vi "MNIST_weight_2color_print_sub.vi"(1 "최소값":dbl=-2.4903133, 2 "최대값":dbl=1.9686242, 3 "배열":dbl[][](array[numeric])=[[0.06671473, 0.012806132, 0.0, 0.007022038, 0.075053, 0.052519154, 0.06788373, 0.058529492, 0.068049595, 0.005657882, 0.0, 0.019000702, 0.10409468, 0.038491603, 0.0, 0.0, 0.0, 0.0, 0.0, 0.0, 0.029719673, 0.0589787, 0.012006044, 0.0, 0.0, 0.0, 0.003024332, 0.0], [0.046028584, 0.084819525, 0.0, 0.0, 0.0, 0.0, 0.027638003, 0.11720828, 0.1663973, 0.25961968, 0.31170687, 0.5143633, 0.3731328, 0.48274365, 0.3280385, 0.40694475, 0.35356778, 0.38455793, 0.24461184, 0.29286602, 0.4148841, 0.408167, 0.36261445, 0.4037632, 0.013449289, 0.07692665, 0.0, 0.028387021], [0.003123008, 0.07717365, 0.07922222, 0.3189904, 0.28332156, 0.062017616, 0.13301574, 0.2924652, 0.2965881, 0.29845756, 0.5972768, 0.6319597, 0.66892195, 0.64722604, 0.62055475, 0.6523688, 0.6531713, 0.83753306, 0.55209464, 0.5967644, 0.49876857, 0.44684905, 0.4477752, 0.5052764, 0.0, 0.0, 0.05617176, 0.020920113], [0.024063304, 0.056840383, 0.0, 0.39337757, 0.30629715, 0.37364787, 0.34470925, 0.5042887, 0.4251124, 0.506105, 0.89726394, 1.1779351, 1.5517938, 1.5492246, 1.8865724, 1.8361284, 1.6005924, 0.8755611, 0.17848553, 0.19548813, 0.6069504, 0.6787907, 0.27294815, 0.20360427, 0.16959353, 0.022720885, 0.0, 0.004873298], [0.08592967, 0.06972434, 0.0, 0.25001055, 0.006792835, 0.4052463, 0.57627326, 1.0514435, 1.1154656, 1.5954032, 1.678078, 0.962688, 0.9687104, 0.89993167, 0.7828392, 1.0242023, 1.1486256, 1.0977578, 0.95435023, 2.3045535, 2.3393528, 2.0629787, 1.3075817, 1.1000681, 0.6505148, 0.15433559, 0.12817676, 0.07914265], [0.07988503, 0.0, 0.0, 0.31504992, 0.37430423, 0.88769066, 1.5406835, 0.6172341, 0.29620916, 0.47488296, 0.26253828, 0.0, 0.0, 0.0, 0.19108367, 0.08104278, 0.515581, 0.37645754, 0.33281028, 0.25179097, 0.22456875, 0.4467277, 0.6797482, 2.2890959, 1.863171, 0.833423, 0.43375036, 0.10676513], [0.0, 0.21307647, 0.5049865, 0.45892584, 0.85746795, 1.20627, 0.48567757, 0.30300915, 0.2370981, 0.0, 0.0, 0.0, 0.0, 0.0, 0.0, 0.0, 0.0, 0.0, 0.0, 0.0, 0.0, 0.054976966, 0.33023435, 0.74540865, 0.82584643, 0.3999863, 0.7573047, 0.37040982], [0.0, 0.48237345, 0.60469353, 0.83249414, 1.066871, 0.8326912, 0.3114878, 0.39401188, 0.03141666, 0.0, 0.0, 0.0, 0.0, 0.0, 0.0, 0.0, 0.0, 0.0, 0.0, 0.0, 0.0, 0.0, 0.1001043, 0.222988, 0.7484905, 0.8096203, 0.9580958, 0.50581247], [0.23312153, 0.81503505, 0.93997633, 0.89034003, 0.5627975, 0.27621332, 0.0881613, 0.30927205, 0.0, 0.0990191, 0.040483538, 0.15247008, 0.17033584, 0.0, 0.0, 0.0, 0.0, 0.0, 0.0, 0.0, 0.095491596, 0.0, 0.15988904, 0.4184175, 0.5088815, 0.7918951, 0.9527885, 0.27583468], [0.34983167, 0.5911077, 1.0430478, 0.4566845, 0.40939477, 0.05266172, 0.0, 0.0, 0.0, 0.02691007, 0.0, 0.016026955, 0.0, 0.0, 0.0, 0.0, 0.009803846, 0.0, 0.0, 0.04322388, 0.032798484, 0.23765023, 0.17197067, 0.44923514, 0.4066683, 0.8139697, 0.9593992, 0.4893604], [0.2907163, 0.5717058, 1.0163774, 0.38863152, 0.29278657, 0.0, 0.0, 0.0, 0.0, 0.0, 0.0, 0.0, 0.0, 0.14446034, 0.09155477, 0.14909427, 0.024265863, 0.0, 0.0, 0.06254616, 6.79e-05, 0.082516626, 0.13715447, 0.32466382, 0.7280415, 0.36880082, 0.9140208, 0.4657428], [0.33525127, 0.6217594, 0.82226497, 0.44135088, 0.16826938, 0.0, 0.0, 0.0, 0.0, 0.0, 0.0, 0.0, 0.011187709, 0.11938254, 0.015615412, 0.0, 0.0, 0.0, 0.0, 0.0, 0.0, 0.0, 0.0, 0.2770026, 0.6325938, 0.631355, 0.6114226, 0.3128235], [0.22835304, 0.7955853, 0.71307003, 0.35154894, 0.0, 0.0, 0.0, 0.0, 0.0, 0.0, 0.0, 0.0, 0.2698419, 0.0, 0.0, 0.0, 0.0, 0.0, 0.0, 0.0, 0.0, 0.0, 0.0, 0.0, 1.0116065, 1.7317381, 0.8858002, 0.3161338], [0.18020941, 0.53125805, 0.6827323, 0.21136676, 0.0, 0.0, 0.0, 0.0, 0.0, 0.0, 0.0, 0.055699844, 0.27314368, 0.0, 0.0, 0.0, 0.0, 0.0, 0.0, 0.0, 0.0, 0.0, 0.0, 0.29844484, 1.5662781, 1.1574728, 0.55202866, 0.085822225], [0.31430015, 0.3546583, 0.7948181, 0.0, 0.0, 0.058352455, 0.0, 0.0, 0.0, 0.0, 0.0, 0.051398423, 0.12864865, 0.0, 0.0, 0.0, 0.0, 0.0, 0.0, 0.0, 0.0, 0.0, 0.016005708, 0.70366126, 1.9256966, 0.7303306, 0.322807, 0.04477008], [0.2970737, 0.0, 0.9035585, 0.04951164, 0.001701124, 0.0, 0.0, 0.009708367, 0.0, 0.09480543, 0.0, 0.0, 0.07521264, 0.11005654, 0.10118085, 0.0, 0.0, 0.0, 0.0, 0.0, 0.0, 0.003710072, 0.018180061, 0.6137533, 1.6424786, 0.8153885, 0.11793761, 0.3056317], [0.29503796, 0.17651856, 0.58721036, 0.18996832, 0.008066228, 0.0, 0.15021098, 0.0, 0.0, 0.18720058, 0.0, 0.0, 0.05664227, 0.12680227, 0.091266185, 0.0, 0.0, 0.0, 0.0, 0.14982839, 0.15584202, 0.2898715, 0.03922329, 0.4780351, 1.6513777, 1.2352444, 0.48265705, 0.5113582], [0.042506717, 0.319817, 0.5209567, 0.3233532, 0.53686345, 0.36480454, 0.19566067, 0.0, 0.0, 0.0, 0.0, 0.0, 0.0, 0.09237474, 0.010339986, 0.0, 0.0, 0.0, 0.012240005, 0.04897488, 0.14640339, 0.19739835, 0.28918922, 0.5824203, 1.4695345, 0.6496217, 0.4080505, 0.47764888], [0.0, 0.2749003, 0.5060507, 0.59561384, 0.82417494, 0.56122655, 0.13255721, 0.04494526, 0.08564969, 0.16170388, 0.0, 0.0, 0.28955424, 0.25209564, 0.0, 0.0, 0.07394005, 0.0, 0.16412586, 0.12713751, 0.0417476, 0.2978168, 0.27767536, 0.7567341, 1.5418999, 0.675374, 0.66687757, 0.3468876], [0.0, 0.41774225, 1.0719318, 0.5180834, 0.65000916, 0.48373982, 0.18409592, 0.0, 0.18066232, 0.44167724, 0.21451446, 0.3340605, 0.2556067, 0.14536966, 0.17981717, 0.17562614, 0.12162264, 0.16115464, 0.23022401, 0.05762116, 0.051491685, 0.2887901, 0.37232834, 0.5140671, 0.8623661, 0.37336326, 0.38255432, 0.26215634], [0.083229735, 0.32688043, 0.608484, 0.41744143, 0.35103565, 0.22907315, 0.3805041, 0.46601966, 0.22916281, 0.5590473, 0.7263584, 0.6074327, 0.49197128, 0.24120732, 0.25589103, 0.28733763, 0.14443557, 0.14488553, 0.30391267, 0.15375902, 0.2781434, 0.5131602, 0.28703067, 0.30208346, 0.0, 0.0, 0.4837919, 0.002000345], [0.0, 0.32385758, 0.6328315, 0.80099195, 0.09775448, 0.07027386, 0.28887808, 0.2724674, 0.1625694, 0.0911344, 0.17027673, 0.32092783, 0.3155498, 0.26486373, 0.20463067, 0.17560713, 0.17749313, 0.29315472, 0.30376917, 0.29634923, 0.20721531, 0.13367781, 0.3279665, 0.28131253, 0.0, 0.020289743, 0.46843135, 0.027426496], [0.023119988, 0.06934198, 0.8942446, 0.27544105, 0.0, 0.28844702, 0.2773134, 0.26331362, 0.0, 0.0, 0.0, 0.0, 0.0, 0.075903945, 0.0, 0.22662191, 0.09397208, 0.24400133, 0.3108672, 0.43392682, 0.11429301, 0.15109178, 0.0, 0.0, 0.0, 0.030385807, 0.6572772, 0.0], [0.0, 0.0, 0.6131038, 0.18363582, 0.53004444, 0.26058108, 0.3353729, 0.16197264, 0.0, 0.1378254, 0.0, 0.054289043, 0.04886698, 0.07301120999999999, 0.004955645, 0.09871276, 0.16584411, 0.08512352, 0.16866887, 0.067276314, 0.0, 0.0, 0.0, 0.0, 0.0, 0.3628522, 0.4819391, 0.07737013], [0.0, 0.0, 0.39253348, 0.7897061, 0.08062354, 0.0, 0.0, 0.0, 0.0, 0.26711848, 0.03603759, 0.21447945, 0.15494835, 0.31901473, 0.26902923, 0.05804711, 0.076432385, 0.0, 0.01643955, 0.047397494, 0.0, 0.0, 0.0, 0.0, 0.23149125, 0.5096788, 0.36468777, 0.001521751], [0.0, 0.0, 0.0, 0.79396546, 0.0, 0.0, 0.0, 0.0, 0.0, 0.0, 0.0, 0.0, 0.0, 0.0, 0.0, 0.0, 0.0, 0.0, 0.0, 0.0, 0.0, 0.0, 0.009036388, 0.0, 0.26618186, 0.32190132, 0.31863904, 0.017361872], [0.041013133, 0.0, 0.012243457, 0.0, 0.0, 0.0, 0.0, 0.0, 0.0, 0.0, 0.0, 0.0, 0.0, 0.0, 0.0, 0.0, 0.0, 0.0, 0.0, 0.0, 0.0, 0.0, 0.0, 0.0, 0.0, 0.17493449, 0.0, 0.070362106], [0.022377841, 0.0, 0.07457931, 0.0, 0.4583214, 0.47468448, 0.0, 0.0, 0.0, 0.0, 0.0, 0.004390556, 0.0, 0.81566125, 0.0, 0.018186547, 0.18291555, 0.5620862, 0.06693945, 0.33189088, 0.0, 0.16514577, 0.3425562, 0.43024477, 0.0, 0.069507696, 0.0, 0.039162096], [0.3611892, 0.0, 0.0, 0.0, 0.0, 0.0, 0.0, 0.0, 0.0, 0.0, 0.0, 0.0, 0.0, 0.0, 0.0, 0.0, 0.0, 0.0, 0.0, 0.0, 0.0, 0.0, 0.0, 0.0, 0.0, 0.0, 0.0, 0.0]]) -> (0 "MNIST_Input":dbl[][](graph)=[[0.06671473, 0.012806132, 0.0, 0.007022038, 0.075053, 0.052519154, 0.06788373, 0.058529492, 0.068049595, 0.005657882, 0.0, 0.019000702, 0.10409468, 0.038491603, 0.0, 0.0, 0.0, 0.0, 0.0, 0.0, 0.029719673, 0.0589787, 0.012006044, 0.0, 0.0, 0.0, 0.003024332, 0.0], [0.046028584, 0.084819525, 0.0, 0.0, 0.0, 0.0, 0.027638003, 0.11720828, 0.1663973, 0.25961968, 0.31170687, 0.5143633, 0.3731328, 0.48274365, 0.3280385, 0.40694475, 0.35356778, 0.38455793, 0.24461184, 0.29286602, 0.4148841, 0.408167, 0.36261445, 0.4037632, 0.013449289, 0.07692665, 0.0, 0.028387021], [0.003123008, 0.07717365, 0.07922222, 0.3189904, 0.28332156, 0.062017616, 0.13301574, 0.2924652, 0.2965881, 0.29845756, 0.5972768, 0.6319597, 0.66892195, 0.64722604, 0.62055475, 0.6523688, 0.6531713, 0.83753306, 0.55209464, 0.5967644, 0.49876857, 0.44684905, 0.4477752, 0.5052764, 0.0, 0.0, 0.05617176, 0.020920113], [0.024063304, 0.056840383, 0.0, 0.39337757, 0.30629715, 0.37364787, 0.34470925, 0.5042887, 0.4251124, 0.506105, 0.89726394, 1.1779351, 1.5517938, 1.5492246, 1.8865724, 1.8361284, 1.6005924, 0.8755611, 0.17848553, 0.19548813, 0.6069504, 0.6787907, 0.27294815, 0.20360427, 0.16959353, 0.022720885, 0.0, 0.004873298], [0.08592967, 0.06972434, 0.0, 0.25001055, 0.006792835, 0.4052463, 0.57627326, 1.0514435, 1.1154656, 1.5954032, 1.678078, 0.962688, 0.9687104, 0.89993167, 0.7828392, 1.0242023, 1.1486256, 1.0977578, 0.95435023, 2.3045535, 2.3393528, 2.0629787, 1.3075817, 1.1000681, 0.6505148, 0.15433559, 0.12817676, 0.07914265], [0.07988503, 0.0, 0.0, 0.31504992, 0.37430423, 0.88769066, 1.5406835, 0.6172341, 0.29620916, 0.47488296, 0.26253828, 0.0, 0.0, 0.0, 0.19108367, 0.08104278, 0.515581, 0.37645754, 0.33281028, 0.25179097, 0.22456875, 0.4467277, 0.6797482, 2.2890959, 1.863171, 0.833423, 0.43375036, 0.10676513], [0.0, 0.21307647, 0.5049865, 0.45892584, 0.85746795, 1.20627, 0.48567757, 0.30300915, 0.2370981, 0.0, 0.0, 0.0, 0.0, 0.0, 0.0, 0.0, 0.0, 0.0, 0.0, 0.0, 0.0, 0.054976966, 0.33023435, 0.74540865, 0.82584643, 0.3999863, 0.7573047, 0.37040982], [0.0, 0.48237345, 0.60469353, 0.83249414, 1.066871, 0.8326912, 0.3114878, 0.39401188, 0.03141666, 0.0, 0.0, 0.0, 0.0, 0.0, 0.0, 0.0, 0.0, 0.0, 0.0, 0.0, 0.0, 0.0, 0.1001043, 0.222988, 0.7484905, 0.8096203, 0.9580958, 0.50581247], [0.23312153, 0.81503505, 0.93997633, 0.89034003, 0.5627975, 0.27621332, 0.0881613, 0.30927205, 0.0, 0.0990191, 0.040483538, 0.15247008, 0.17033584, 0.0, 0.0, 0.0, 0.0, 0.0, 0.0, 0.0, 0.095491596, 0.0, 0.15988904, 0.4184175, 0.5088815, 0.7918951, 0.9527885, 0.27583468], [0.34983167, 0.5911077, 1.0430478, 0.4566845, 0.40939477, 0.05266172, 0.0, 0.0, 0.0, 0.02691007, 0.0, 0.016026955, 0.0, 0.0, 0.0, 0.0, 0.009803846, 0.0, 0.0, 0.04322388, 0.032798484, 0.23765023, 0.17197067, 0.44923514, 0.4066683, 0.8139697, 0.9593992, 0.4893604], [0.2907163, 0.5717058, 1.0163774, 0.38863152, 0.29278657, 0.0, 0.0, 0.0, 0.0, 0.0, 0.0, 0.0, 0.0, 0.14446034, 0.09155477, 0.14909427, 0.024265863, 0.0, 0.0, 0.06254616, 6.79e-05, 0.082516626, 0.13715447, 0.32466382, 0.7280415, 0.36880082, 0.9140208, 0.4657428], [0.33525127, 0.6217594, 0.82226497, 0.44135088, 0.16826938, 0.0, 0.0, 0.0, 0.0, 0.0, 0.0, 0.0, 0.011187709, 0.11938254, 0.015615412, 0.0, 0.0, 0.0, 0.0, 0.0, 0.0, 0.0, 0.0, 0.2770026, 0.6325938, 0.631355, 0.6114226, 0.3128235], [0.22835304, 0.7955853, 0.71307003, 0.35154894, 0.0, 0.0, 0.0, 0.0, 0.0, 0.0, 0.0, 0.0, 0.2698419, 0.0, 0.0, 0.0, 0.0, 0.0, 0.0, 0.0, 0.0, 0.0, 0.0, 0.0, 1.0116065, 1.7317381, 0.8858002, 0.3161338], [0.18020941, 0.53125805, 0.6827323, 0.21136676, 0.0, 0.0, 0.0, 0.0, 0.0, 0.0, 0.0, 0.055699844, 0.27314368, 0.0, 0.0, 0.0, 0.0, 0.0, 0.0, 0.0, 0.0, 0.0, 0.0, 0.29844484, 1.5662781, 1.1574728, 0.55202866, 0.085822225], [0.31430015, 0.3546583, 0.7948181, 0.0, 0.0, 0.058352455, 0.0, 0.0, 0.0, 0.0, 0.0, 0.051398423, 0.12864865, 0.0, 0.0, 0.0, 0.0, 0.0, 0.0, 0.0, 0.0, 0.0, 0.016005708, 0.70366126, 1.9256966, 0.7303306, 0.322807, 0.04477008], [0.2970737, 0.0, 0.9035585, 0.04951164, 0.001701124, 0.0, 0.0, 0.009708367, 0.0, 0.09480543, 0.0, 0.0, 0.07521264, 0.11005654, 0.10118085, 0.0, 0.0, 0.0, 0.0, 0.0, 0.0, 0.003710072, 0.018180061, 0.6137533, 1.6424786, 0.8153885, 0.11793761, 0.3056317], [0.29503796, 0.17651856, 0.58721036, 0.18996832, 0.008066228, 0.0, 0.15021098, 0.0, 0.0, 0.18720058, 0.0, 0.0, 0.05664227, 0.12680227, 0.091266185, 0.0, 0.0, 0.0, 0.0, 0.14982839, 0.15584202, 0.2898715, 0.03922329, 0.4780351, 1.6513777, 1.2352444, 0.48265705, 0.5113582], [0.042506717, 0.319817, 0.5209567, 0.3233532, 0.53686345, 0.36480454, 0.19566067, 0.0, 0.0, 0.0, 0.0, 0.0, 0.0, 0.09237474, 0.010339986, 0.0, 0.0, 0.0, 0.012240005, 0.04897488, 0.14640339, 0.19739835, 0.28918922, 0.5824203, 1.4695345, 0.6496217, 0.4080505, 0.47764888], [0.0, 0.2749003, 0.5060507, 0.59561384, 0.82417494, 0.56122655, 0.13255721, 0.04494526, 0.08564969, 0.16170388, 0.0, 0.0, 0.28955424, 0.25209564, 0.0, 0.0, 0.07394005, 0.0, 0.16412586, 0.12713751, 0.0417476, 0.2978168, 0.27767536, 0.7567341, 1.5418999, 0.675374, 0.66687757, 0.3468876], [0.0, 0.41774225, 1.0719318, 0.5180834, 0.65000916, 0.48373982, 0.18409592, 0.0, 0.18066232, 0.44167724, 0.21451446, 0.3340605, 0.2556067, 0.14536966, 0.17981717, 0.17562614, 0.12162264, 0.16115464, 0.23022401, 0.05762116, 0.051491685, 0.2887901, 0.37232834, 0.5140671, 0.8623661, 0.37336326, 0.38255432, 0.26215634], [0.083229735, 0.32688043, 0.608484, 0.41744143, 0.35103565, 0.22907315, 0.3805041, 0.46601966, 0.22916281, 0.5590473, 0.7263584, 0.6074327, 0.49197128, 0.24120732, 0.25589103, 0.28733763, 0.14443557, 0.14488553, 0.30391267, 0.15375902, 0.2781434, 0.5131602, 0.28703067, 0.30208346, 0.0, 0.0, 0.4837919, 0.002000345], [0.0, 0.32385758, 0.6328315, 0.80099195, 0.09775448, 0.07027386, 0.28887808, 0.2724674, 0.1625694, 0.0911344, 0.17027673, 0.32092783, 0.3155498, 0.26486373, 0.20463067, 0.17560713, 0.17749313, 0.29315472, 0.30376917, 0.29634923, 0.20721531, 0.13367781, 0.3279665, 0.28131253, 0.0, 0.020289743, 0.46843135, 0.027426496], [0.023119988, 0.06934198, 0.8942446, 0.27544105, 0.0, 0.28844702, 0.2773134, 0.26331362, 0.0, 0.0, 0.0, 0.0, 0.0, 0.075903945, 0.0, 0.22662191, 0.09397208, 0.24400133, 0.3108672, 0.43392682, 0.11429301, 0.15109178, 0.0, 0.0, 0.0, 0.030385807, 0.6572772, 0.0], [0.0, 0.0, 0.6131038, 0.18363582, 0.53004444, 0.26058108, 0.3353729, 0.16197264, 0.0, 0.1378254, 0.0, 0.054289043, 0.04886698, 0.07301120999999999, 0.004955645, 0.09871276, 0.16584411, 0.08512352, 0.16866887, 0.067276314, 0.0, 0.0, 0.0, 0.0, 0.0, 0.3628522, 0.4819391, 0.07737013], [0.0, 0.0, 0.39253348, 0.7897061, 0.08062354, 0.0, 0.0, 0.0, 0.0, 0.26711848, 0.03603759, 0.21447945, 0.15494835, 0.31901473, 0.26902923, 0.05804711, 0.076432385, 0.0, 0.01643955, 0.047397494, 0.0, 0.0, 0.0, 0.0, 0.23149125, 0.5096788, 0.36468777, 0.001521751], [0.0, 0.0, 0.0, 0.79396546, 0.0, 0.0, 0.0, 0.0, 0.0, 0.0, 0.0, 0.0, 0.0, 0.0, 0.0, 0.0, 0.0, 0.0, 0.0, 0.0, 0.0, 0.0, 0.009036388, 0.0, 0.26618186, 0.32190132, 0.31863904, 0.017361872], [0.041013133, 0.0, 0.012243457, 0.0, 0.0, 0.0, 0.0, 0.0, 0.0, 0.0, 0.0, 0.0, 0.0, 0.0, 0.0, 0.0, 0.0, 0.0, 0.0, 0.0, 0.0, 0.0, 0.0, 0.0, 0.0, 0.17493449, 0.0, 0.070362106], [0.022377841, 0.0, 0.07457931, 0.0, 0.4583214, 0.47468448, 0.0, 0.0, 0.0, 0.0, 0.0, 0.004390556, 0.0, 0.81566125, 0.0, 0.018186547, 0.18291555, 0.5620862, 0.06693945, 0.33189088, 0.0, 0.16514577, 0.3425562, 0.43024477, 0.0, 0.069507696, 0.0, 0.039162096], [0.3611892, 0.0, 0.0, 0.0, 0.0, 0.0, 0.0, 0.0, 0.0, 0.0, 0.0, 0.0, 0.0, 0.0, 0.0, 0.0, 0.0, 0.0, 0.0, 0.0, 0.0, 0.0, 0.0, 0.0, 0.0, 0.0, 0.0, 0.0]])   [LabVIEW 2021]
panel:
  in  "색선택 2":u32[](array[colorbox])=[0, 16711680, 65280]
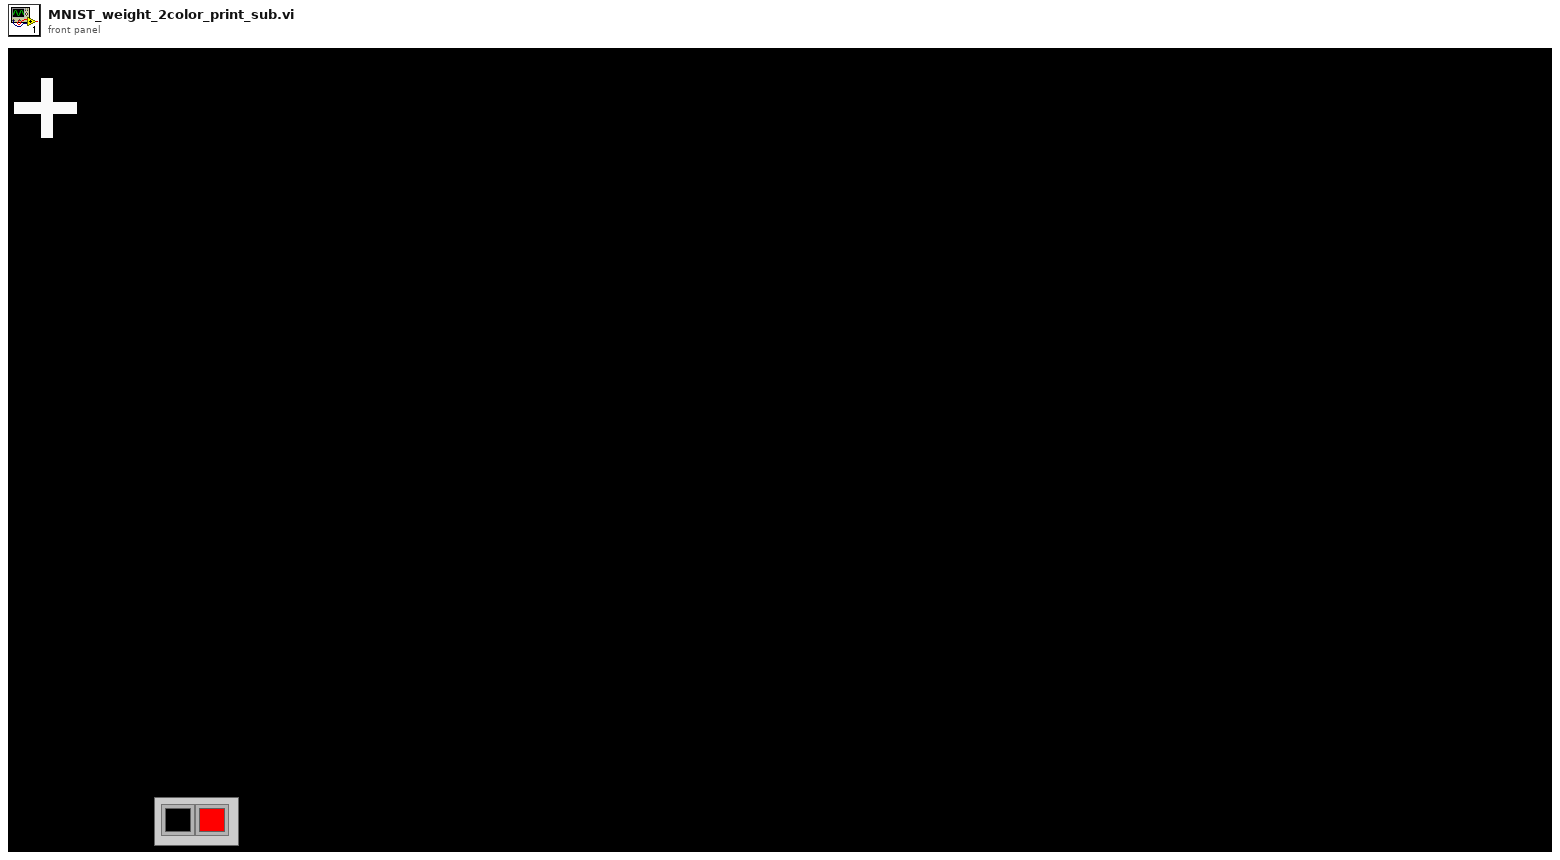
[diagram p1: front panel]
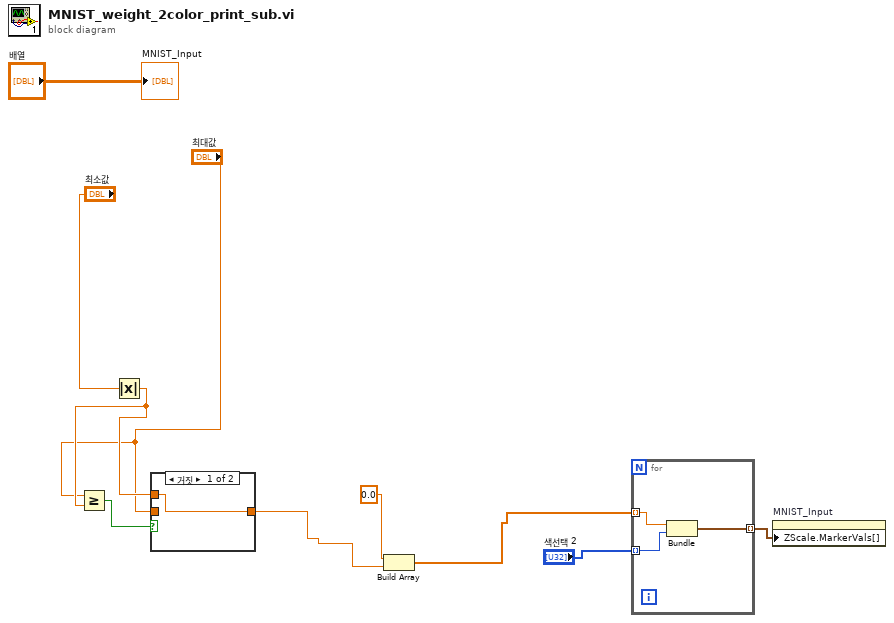
[diagram p0: block diagram]
diagram:
  n1 = Absolute Value(x="최소값") -> (abs(x)=w4:dbl)
  n2 = Greater Or Equal?(x="최대값", y=w4) -> (x >= y?=w7:bool)
  n3 = case shown="거짓" w7 {
    tunnel: "최대값" -> [_ w12]
    tunnel: [w11 w12] -> w1
    tunnel: w4 -> [w11 _]
    frame False {
    }
    frame True {
    }
  }
  n4 = Build Array(0.0 ("원소"), w1) -> (w5:dbl[])
  n5 = for {
    tunnel: w5 -> [w15] mode=indexing
    tunnel: "색선택 2" -> [w14] mode=indexing
    tunnel: [w13] -> w9 mode=indexing
    n6 = Bundle("최대값"=w15, "색 상자"=w14) -> (w13:cluster{"최대값":dbl, "색 상자":u32})  [unwired: 1 in]
  }
  n7 = property on="MNIST_Input" class="IntGraph (엄격한)"("ZScale.MarkerVals[]"=w9) -> ()  [unwired: 2 in, 2 out]
  "MNIST_Input" <- "배열"
